vi "v0.2_son_http.vi"(8 "error in":errorcluster, 10 "ServoON":bool, 11 "mbed.lvclass IN":refnum<class "mbed.lvclass">) -> (0 "error out":errorcluster, 3 "mbed.lvclass OUT":refnum<class "mbed.lvclass">)   [LabVIEW 2011]
doc: "<B>Servo ON</B>\n\nEncender/Apagar el servomotor utilizando una variable boolena"
uses:
  C:/mbed/Transport Mechanisms/mbed/mbed.lvclass
  C:/mbed/mbed Interface/RPCFunction/RPCFunction.lvclass
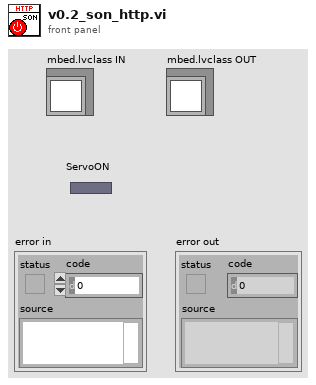
[diagram p1: front panel]
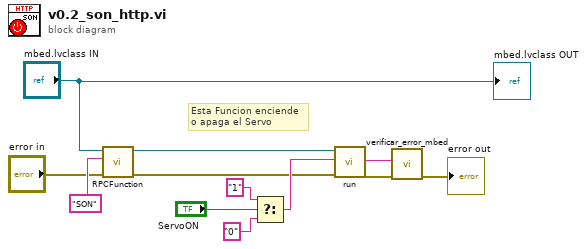
[diagram p0: block diagram]
diagram:
  # "Esta Funcion enciende\no apaga el Servo"
  n1 = call "RPCFunction.vi"("error in (no error)"="error in", "Existing Obj Name"="SON", "mbed_LVLibrary.lvlib:mbed.lvclass"="mbed.lvclass IN") -> ("error out"=w1:errorcluster, "mbed_LVLibrary.lvlib:Packet.lvclass 2"=w11:refnum<class "RPCFunction.lvclass">)  [unwired: 6 in, 1 out]
  n2 = Select(t="1", s="ServoON", f="0") -> (s? t:f=w9:string)
  n3 = call "run.vi"("error in (no error)"=w1, "Input"=w9, "Packet in"=w11) -> ("error out"=w4:errorcluster, "Output"=w5:string)  [unwired: 6 in, 1 out]
  n4 = call "verificar_error_mbed.vi"("error in (no error)"=w4, "desde_mbed"=w5) -> ("error out"=→"error out":errorcluster)  [unwired: 8 in, 1 out]
  "mbed.lvclass OUT" <- "mbed.lvclass IN"
